vi "Delete Type Tags.vi"() -> ()   [LabVIEW 2021]
uses:
  <vilib>/Utility/traverseref.llb/TRef TravTarget.ctl
  <vilib>/Utility/traverseref.llb/VI Scripting - Traverse.lvlib
panel:
  out "Array":string[](array[string])
  out "size(s)":i32
  out "error out":errorcluster
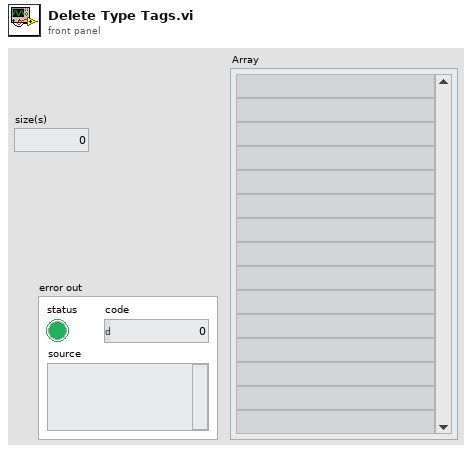
[diagram p1: front panel]
types:
  T1 = typedef "TRef TravTarget.ctl" = enum16{"FP", "BD", "Other"}
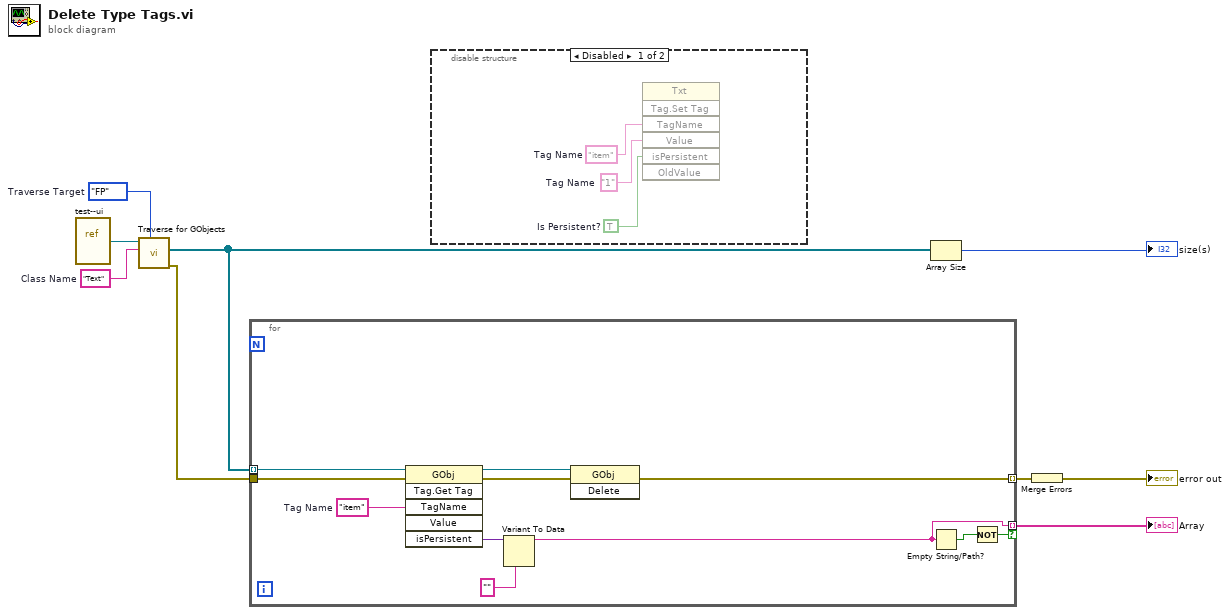
[diagram p0: block diagram]
diagram:
  w8 = TRef_TravTarget."FP"  # Traverse Target
  w9 = "Text"  # Class Name
  n1 = vi-ref "test--ui.vi"() -> (w5:refnum<vi>)
  n2 = call <vilib>:"Traverse for GObjects.vi"("Traverse Target"=w8, "Class Name"=w9, "VI Refnum"=w5) -> ("error out"=w3:errorcluster, "References"=w6:refnum<vi>[])  [unwired: 5 in, 2 out]
  n3 = for {
    tunnel: w6 -> [w19] mode=indexing
    tunnel: [w14] -> w4 mode=indexing if=w15
    tunnel: w3 -> [w13]
    tunnel: [w11] -> w2 mode=indexing
    w20 = "item"  # Tag Name
    n4 = invoke class="GObj" method="Tag.Get Tag"(reference=w19, error in=w13, "TagName"=w20) -> (reference out=w10:refnum<vi>, error out=w12:errorcluster, "isPersistent"=w18:variant)  [unwired: 3 in, 3 out]
    n5 = Variant To Data(type="", Variant=w18) -> (data=w14:string)  [unwired: 1 in, 1 out]
    n6 = invoke class="GObj" method="Delete"(reference=w10, error in=w12) -> (error out=w11:errorcluster)  [unwired: 1 in, 2 out]
    n7 = Empty String/Path?(string/path=w14) -> (empty?=w16:bool)
    n8 = Not(x=w16) -> (.not. x?=w15:bool)
  }
  "Array" <- w4
  n9 = disable-structure shown="Disabled" {
    frame Disabled {
      w25 = TRUE  # Is Persistent?
      w24 = "1"  # Tag Name
      w23 = "item"  # Tag Name
      n10 = invoke class="Txt" method="Tag.Set Tag"("TagName"=w23, "Value"=w24, "isPersistent"=w25) -> (reference=w22:refnum<vi>, error in=w21:errorcluster)  [unwired: 2 in, 7 out]
    }
    frame Enabled {
    }
  }
  n11 = Array Size(array=w6) -> (size(s)=→"size(s)":i32)
  n12 = Merge Errors(w2) -> (→"error out":errorcluster)
